vi "CorruptIconErrorMessage.vi"() -> (0 "corruptIconErrorMsg":string="The following files produced errors on load:")   [LabVIEW 2020]
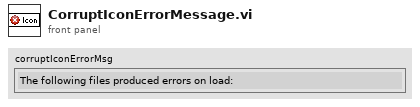
[diagram p1: front panel]
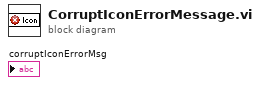
[diagram p0: block diagram]
diagram:
